vi "Sellmeier_control_stage.vi"() -> ()   [LabVIEW 2018]
uses:
  <vilib>/express/express arith-compare/Formula/XNode/ExpressFormulaBlockNode.xnode
  DLL/XMT_DLL_SER.dll
panel:
  out "RData":sgl
  in  "电机安装偏差角度":dbl
  in  "停止":bool
  in  "Ch":u8
  in  "Address":u8=1
  in  "ReFlag 4":u8
  out "SHG theta":dbl
  out "lam_idler(o) (nm)":dbl
  out "lam_shg(e) (nm)":dbl
  in  "lam_signal(nm)":dbl
  in  "COM":u64=3
  out "int":i8
  out "返回类型":u8
  out "错误输出":errorcluster
  # "需要给输入信号加个范围"
  # "开环O:79"
  # "闭环C:67"
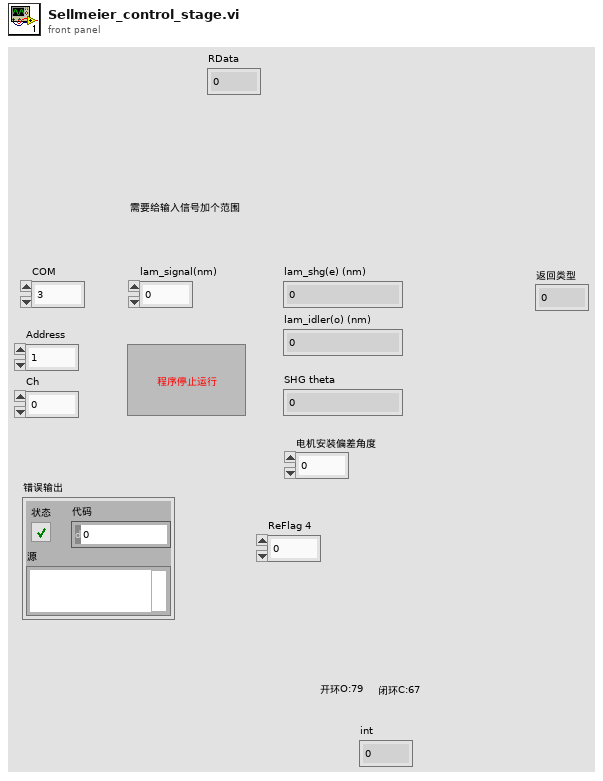
[diagram p1: front panel]
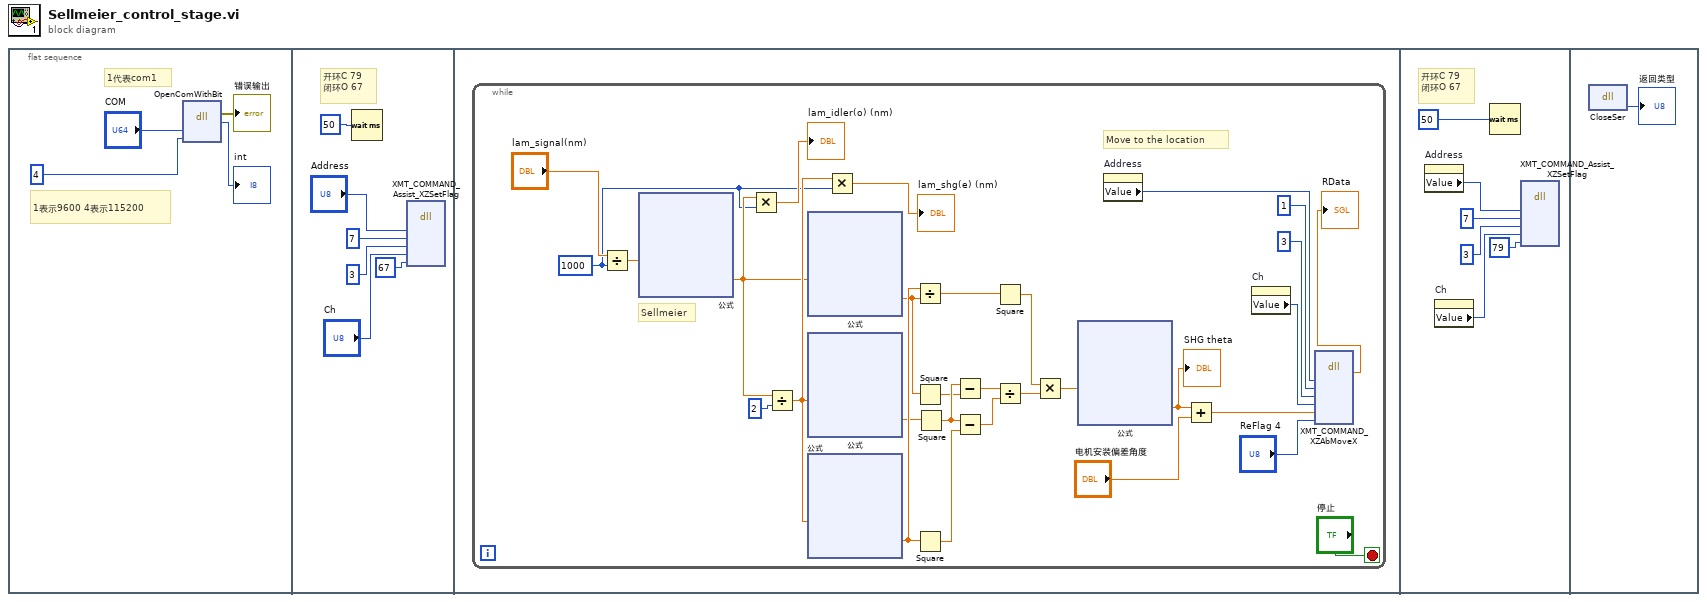
[diagram p0: block diagram]
diagram:
  n1 = flat-sequence {
    frame #0 {
      # "1表示9600 4表示115200"
      # "1代表com1"
      n2 = dll-call lib="C:/Users/cy3486/OneDrive/Desktop/OPO_control_scripts/SHG_motor_control/DLL/XMT_DLL_SER.dll" fn="OpenComWithBit"("m_com"="COM", "BaudRate"=u8 4) -> (error out=→"错误输出":errorcluster, "int"=→"int":i8)  [unwired: 5 in, 1 out]
    }
    frame #1 {
      # "开环C 79\n闭环O 67"
      n3 = Wait (ms)(milliseconds to wait=u32 50 ("等待时间（毫秒）")) -> ()  [unwired: 1 out]
      n4 = dll-call lib="C:/Users/cy3486/OneDrive/Desktop/OPO_control_scripts/SHG_motor_control/DLL/XMT_DLL_SER.dll" fn="XMT_COMMAND_Assist_XZSetFlag"("Address"="Address", "Command_B3"=u16 7, "Command_B4"=u16 3 ("Command_B3"), "Ch"="Ch", "SetFalg"=67) -> ()  [unwired: 9 in, 2 out]
    }
    frame #2 {
      n5 = while {
        stop <- "停止" stop-if-true
        w16 = 1000
        # "Move to the location"
        # "Sellmeier"
        n6 = Divide(x="lam_signal(nm)", y=w16) -> (x/y=w32:dbl)
        n7 = xnode "公式"("lam"=w32) -> ("结果"=w33:dbl)  [unwired: 1 in, 1 out]
        n8 = Multiply(x=w33, y=w16) -> (x*y=→"lam_idler(o) (nm)":dbl)
        n9 = Divide(x=w33, y=2) -> (x/y=w36:dbl)
        n10 = xnode "公式"("lam"=w33) -> ("结果"=w25:dbl)  [unwired: 1 in, 1 out]
        n11 = xnode "公式"("lam"=w36) -> ("结果"=w21:dbl)  [unwired: 1 in, 1 out]
        n12 = xnode "公式"("lam"=w36) -> ("结果"=w29:dbl)  [unwired: 1 in, 1 out]
        n13 = Multiply(x=w36, y=w16) -> (x*y=→"lam_shg(e) (nm)":dbl)
        n14 = Divide(x=w29, y=w25) -> (x/y=w27:dbl)
        n15 = Square(x=w25) -> (x^2=w20:dbl)
        n16 = Square(x=w29) -> (x^2=w28:dbl)
        n17 = Square(x=w21) -> (x^2=w26:dbl)
        n18 = Subtract(x=w26, y=w20) -> (x-y=w22:dbl)
        n19 = Subtract(x=w26, y=w28) -> (x-y=w23:dbl)
        n20 = Square(x=w27) -> (x^2=w19:dbl)
        n21 = Divide(x=w22, y=w23) -> (x/y=w24:dbl)
        n22 = Multiply(x=w19, y=w24) -> (x*y=w30:dbl)
        n23 = xnode "公式"("X1"=w30) -> ("结果"=w13:dbl)  [unwired: 1 in, 1 out]
        "SHG theta" <- w13
        n24 = property on="Address" class="DigNum (严格)"() -> ("Value"=w38:u8)  [unwired: 2 in, 2 out]
        n25 = Add(x=w13, y="电机安装偏差角度") -> (x+y=w12:dbl)
        n26 = property on="Ch" class="DigNum (严格)"() -> ("Value"=w37:u8)  [unwired: 2 in, 2 out]
        n27 = dll-call lib="C:/Users/cy3486/OneDrive/Desktop/OPO_control_scripts/SHG_motor_control/DLL/XMT_DLL_SER.dll" fn="XMT_COMMAND_XZAbMoveX"("Address"=w38, "Command_B3"=u16 1, "Command_B4"=u16 3 ("Command_B3"), "Ch"=w37, "MoveX_f"=w12, "ReFlag"="ReFlag 4") -> ("RData"=→"RData":sgl)  [unwired: 9 in, 2 out]
      }
    }
    frame #3 {
      # "开环C 79\n闭环O 67"
      n28 = property on="Address" class="DigNum (严格)"() -> ("Value"=w82:u8)  [unwired: 2 in, 2 out]
      n29 = property on="Ch" class="DigNum (严格)"() -> ("Value"=w81:u8)  [unwired: 2 in, 2 out]
      n30 = Wait (ms)(milliseconds to wait=u32 50 ("等待时间（毫秒）")) -> ()  [unwired: 1 out]
      n31 = dll-call lib="C:/Users/cy3486/OneDrive/Desktop/OPO_control_scripts/SHG_motor_control/DLL/XMT_DLL_SER.dll" fn="XMT_COMMAND_Assist_XZSetFlag"("Address"=w82, "Command_B3"=u16 7, "Command_B4"=u16 3 ("Command_B3"), "Ch"=w81, "SetFalg"=79) -> ()  [unwired: 9 in, 2 out]
    }
    frame #4 {
      n32 = dll-call lib="C:/Users/cy3486/OneDrive/Desktop/OPO_control_scripts/SHG_motor_control/DLL/XMT_DLL_SER.dll" fn="CloseSer"() -> ("返回类型"=→"返回类型":u8)  [unwired: 3 in, 2 out]
    }
  }
